vi "StateLED.vi"(0 "Master State In":T1(ring)) -> ()   [LabVIEW 2020]
doc: "This VI manages the apperance of the LEDs. The LED coloration and blink pattern report the robot mode and status. See project documentation for details."
uses:
  <vilib>/Rock Robotics/WPI/DriverStation/WPI_DriverStationRobotMode2.ctl
  GlobalMiscellaneous.vi
  GlobalDriverStationData.vi
  GlobalDrivebase.vi
  GlobalAutonomous.vi
  GlobalPoseAndTargeting.vi
  <vilib>/vision/NI_Vision_Development_Module.lvlib
panel:
  in  "Background":u32(colorbox)=16717311
  in  "Human Control":u32(colorbox)=65280
  in  "Master Caution":u32(colorbox)=16736256
  in  "User Value Choice":u8(slide)=255 step=1 scale=0.0..255.0
  in  "User Saturation Choice":u8(slide)=255 step=1 scale=0.0..255.0
  in  "Pressure Insert":u32(colorbox)=91
  in  "Battery Insert":u32(colorbox)=65282
  in  "Pressure Background":u32(colorbox)=16711680
  in  "Battery Background":u32(colorbox)=16711680
  in  "Pressure LED Length":i32=6
  in  "Battery LED Length":i32=6
  in  "Battery Index":i32=4
  in  "Pressure Index":i32=4
  in  "Swerve 2 LED Index":i32
  in  "Swerve 3 LED Index":i32
  in  "Swerve 0 LED Index":i32=18
  in  "Swerve LED Length":i32=2
  in  "Swerve 1 LED Index":i32=18
  in  "Locate LED":bool
  in  "LED Index":i32
  out "User Blue":u8
  out "User Green":u8=255
  out "User Red":u8
  in  "Choose Hue":bool
  in  "User Hue Choice":u8(slide)=255 step=1 scale=0.0..255.0
  in  "Nominal":u32(colorbox)=65280
  in  "Master Alarm":u32(colorbox)=16711680
  in  "Robot Control":u32(colorbox)=16727040
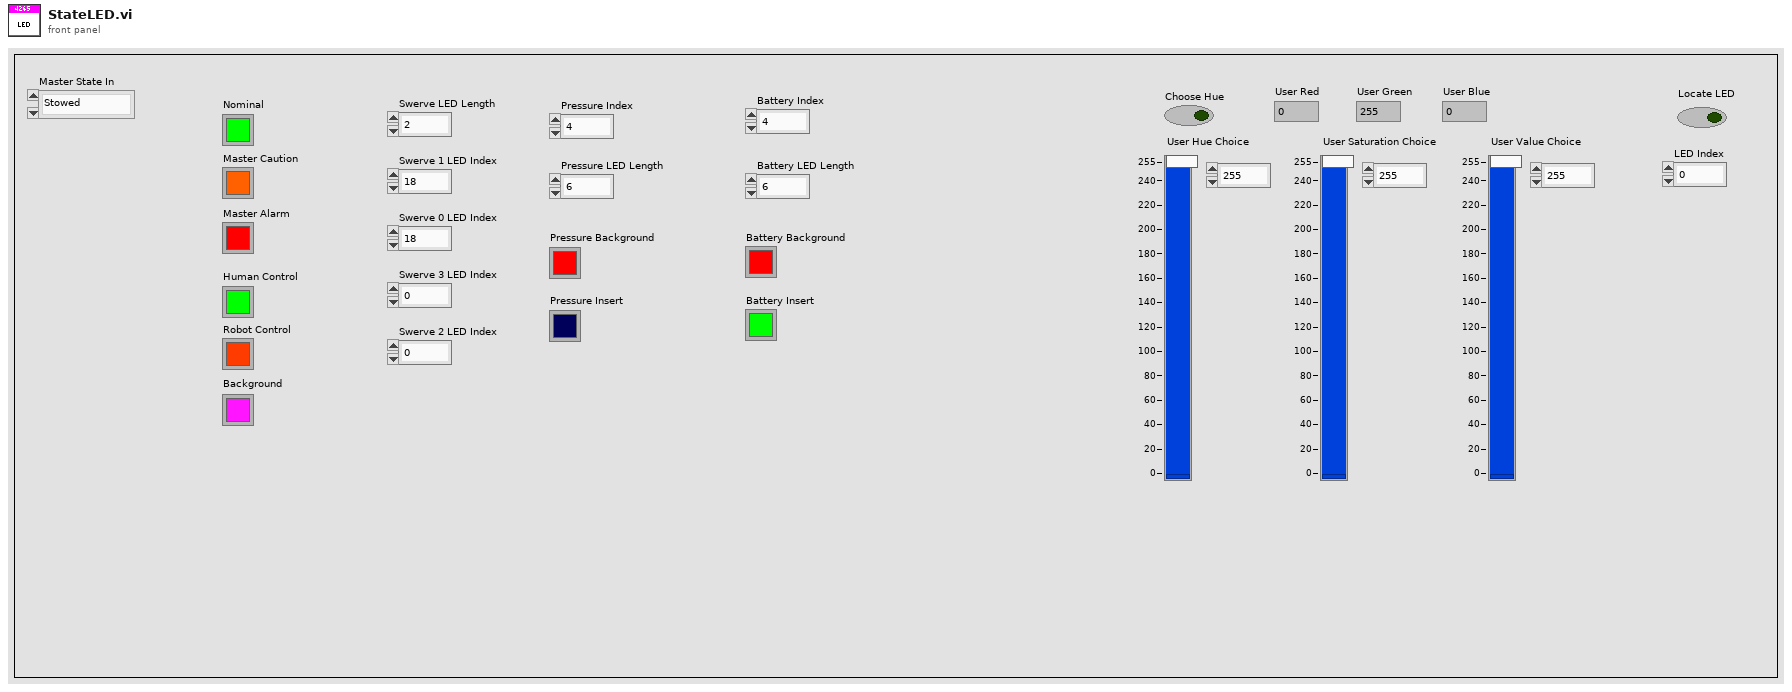
[diagram p1: front panel]
types:
  T1 = enum16{"Stowed", "Balancing", "Scoring", "Hoppering", "Ground", "Shelf"}
  T2 = enum16{"Normal", "Party Mode", "Choose Hue", "Debug", "Locate LED", "Distance Rainbow"}
  T3 = typedef "WPI_DriverStationRobotMode2.ctl" = enum16{"Autonomous Disabled", "Autonomous Enabled", "Teleop Disabled", "Teleop Enabled", "Disconnected", "Finish", "Test Disabled", "Test Enabled", "Emergency Stopped"}
  T4 = enum16{"Low Gear", "High Gear", "Transiting", "Unknown", "Force Low Gear"}
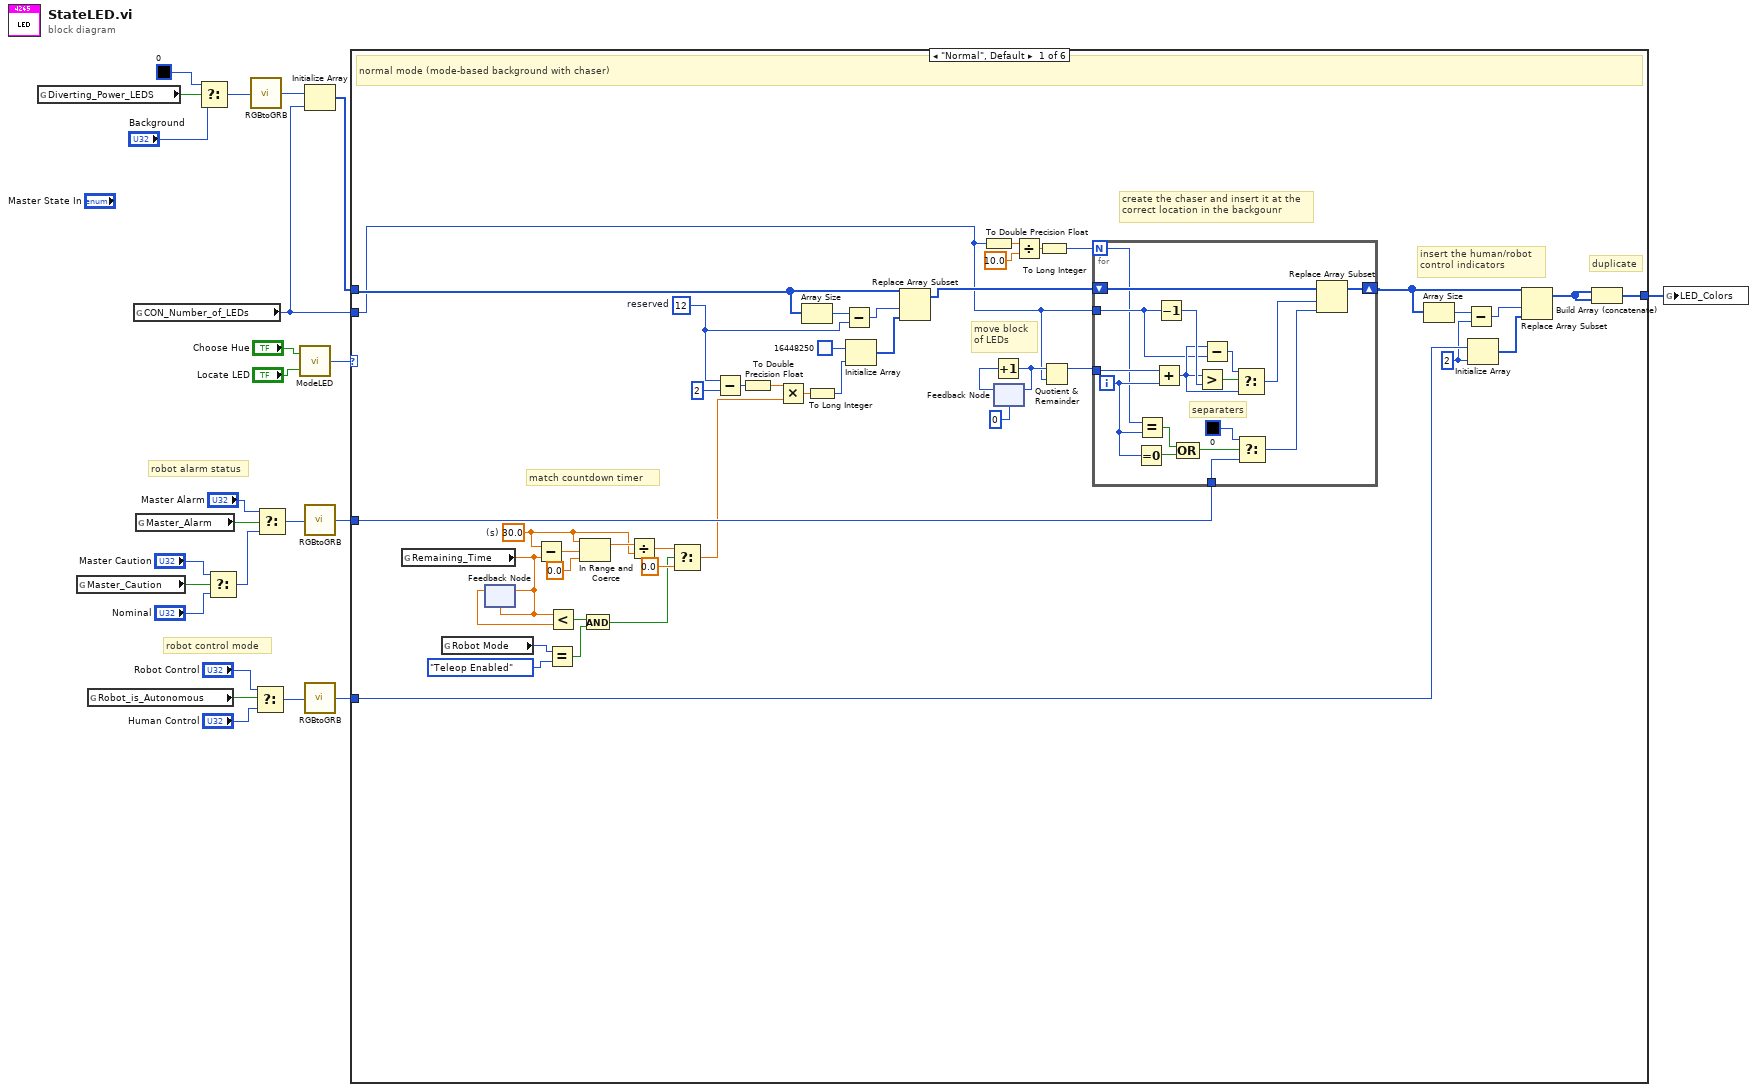
[diagram p0: block diagram]
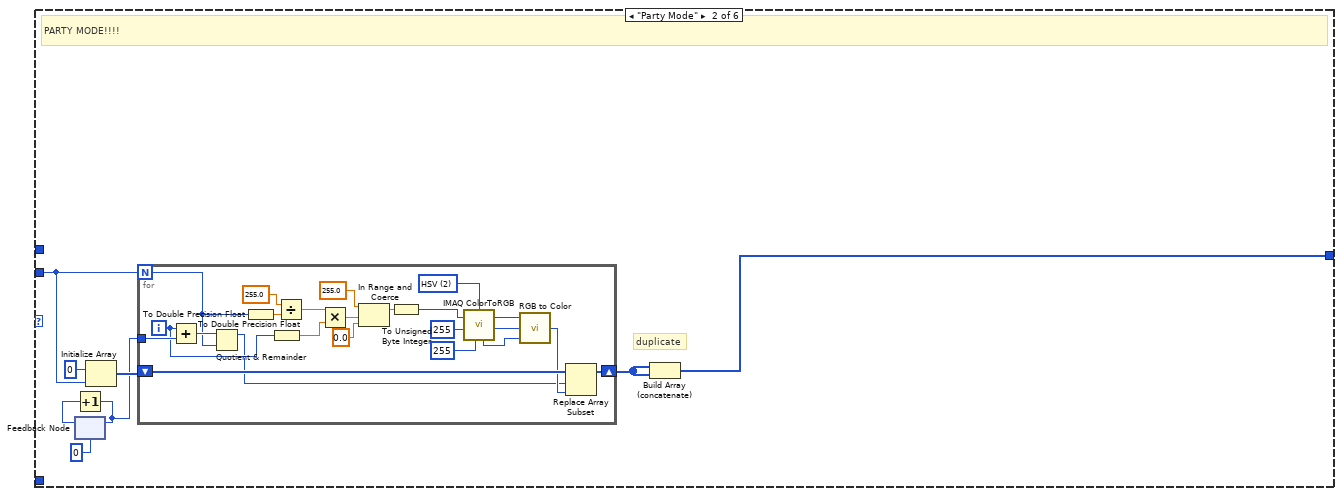
[diagram p2: hidden frame]
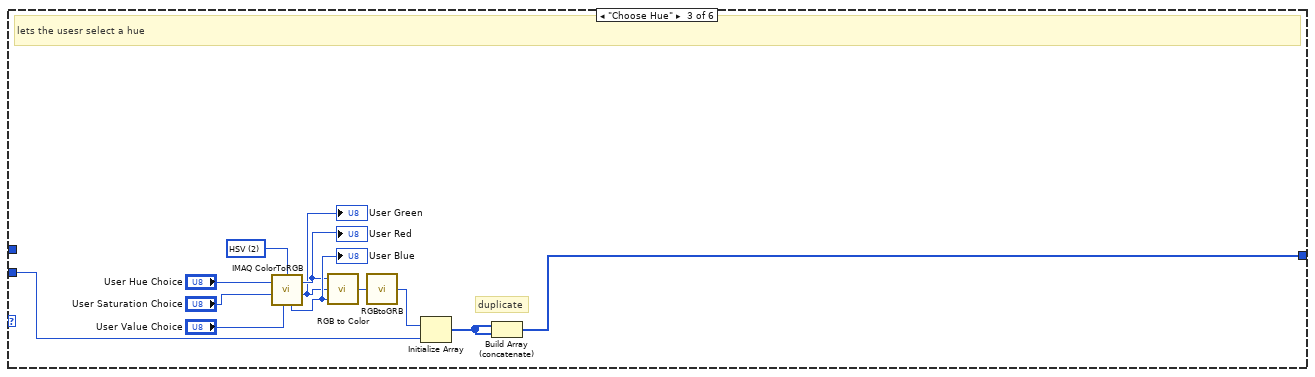
[diagram p3: hidden frame]
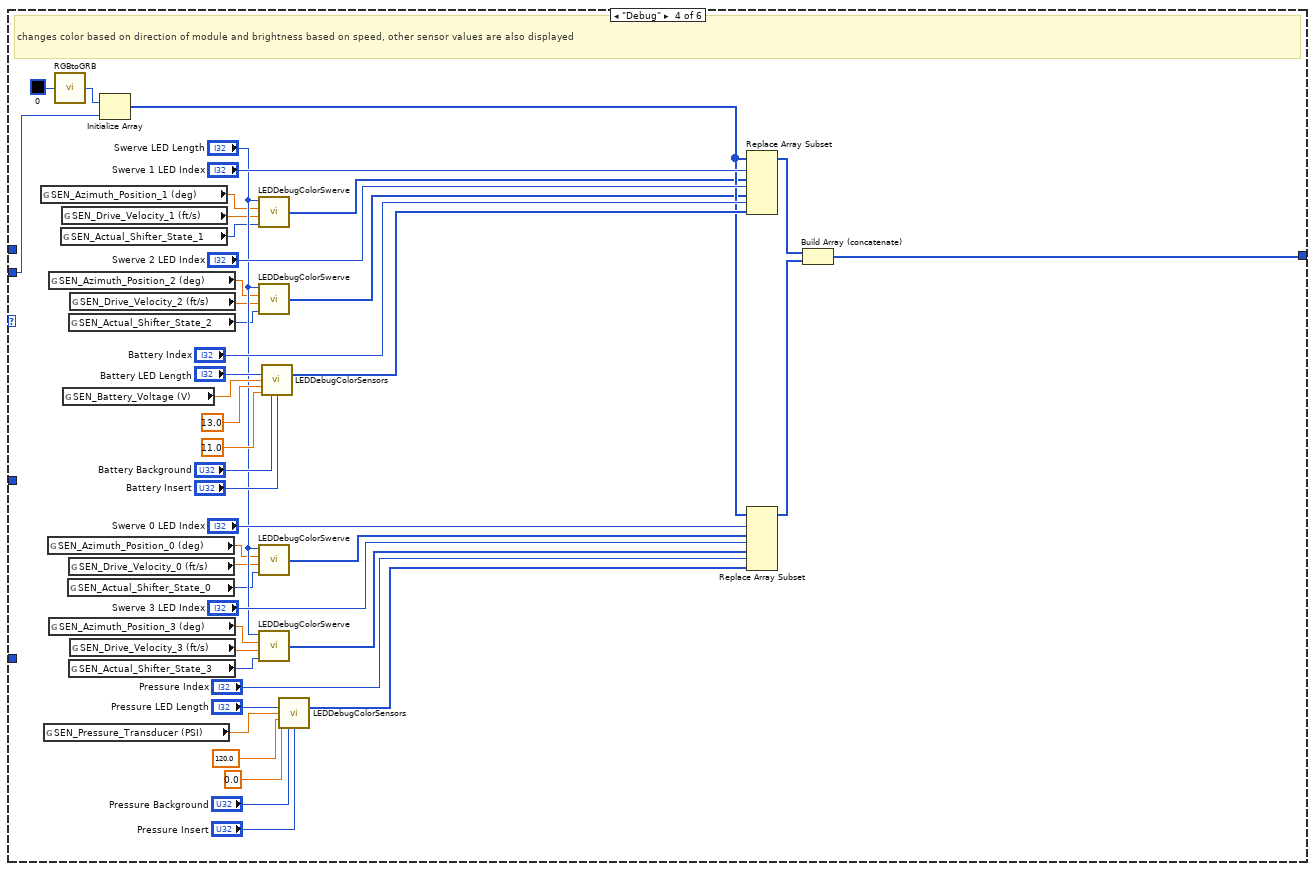
[diagram p4: hidden frame]
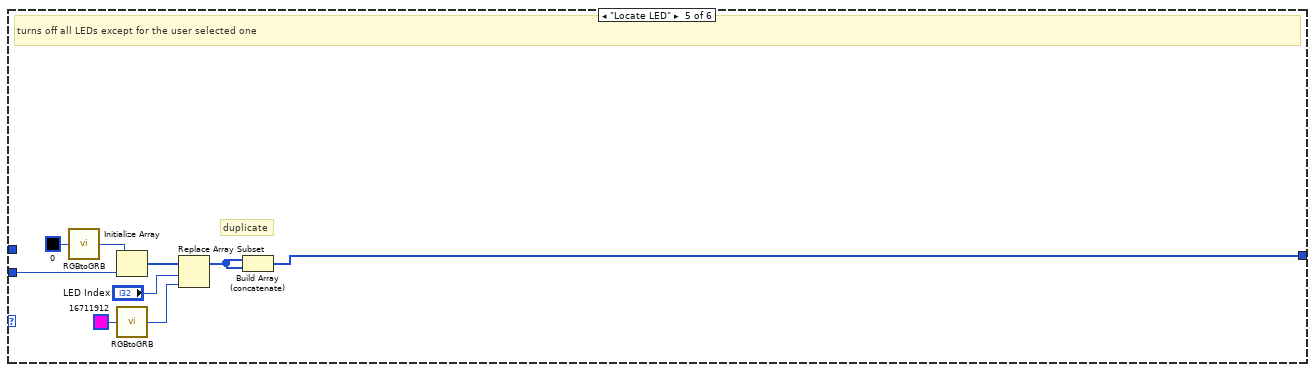
[diagram p5: hidden frame]
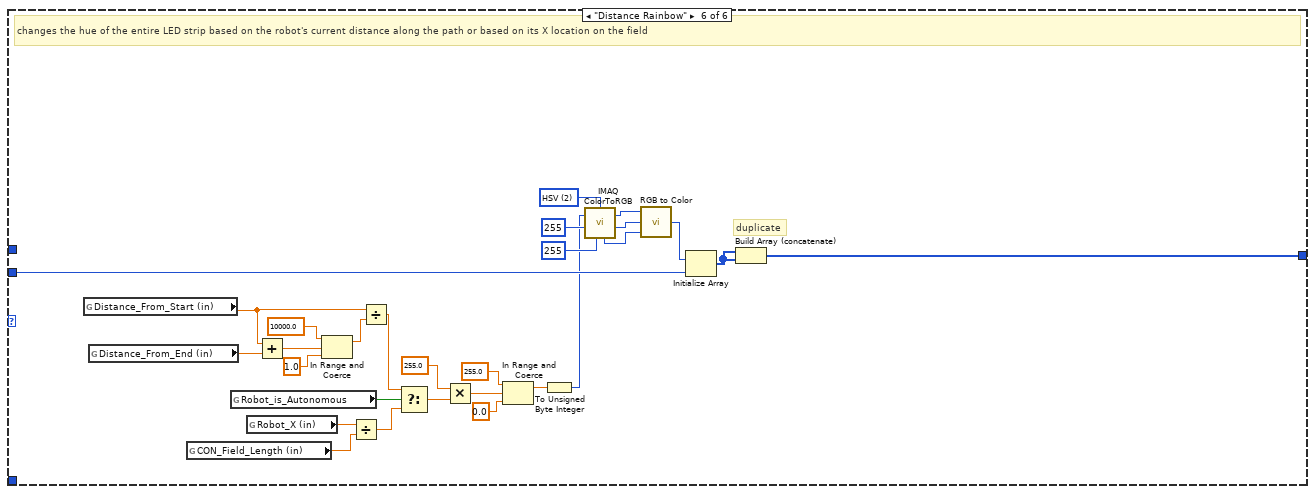
[diagram p6: hidden frame]
diagram:
  # "robot control mode"
  # "robot alarm status"
  n1 = global read "GlobalMiscellaneous.vi" "Diverting_Power_LEDS"() -> (w16:bool)
  n2 = global read "GlobalMiscellaneous.vi" "Master_Caution"() -> (w9:bool)
  n3 = global read "GlobalDriverStationData.vi" "Robot_is_Autonomous"() -> (w14:bool)
  n4 = global read "GlobalMiscellaneous.vi" "CON_Number_of_LEDs"() -> (w1:u16)
  n5 = global read "GlobalMiscellaneous.vi" "Master_Alarm"() -> (w15:bool)
  n6 = Select(t=u32 0 ("Diverting Power"), s=w16, f="Background") -> (s? t:f=w4:u32)
  n7 = Select(t="Master Caution", s=w9, f="Nominal") -> (s? t:f=w8:u32)
  n8 = call "RGBtoGRB.vi"("Color (RGB)"=w4) -> ("Color (GRB)"=w24:u32)
  n9 = Select(t="Robot Control", s=w14, f="Human Control") -> (s? t:f=w13:u32)
  n10 = Select(t="Master Alarm", s=w15, f=w8) -> (s? t:f=w11:u32)
  n11 = call "ModeLED.vi"("Locate LED"="Locate LED", "Choose Hue"="Choose Hue") -> ("LED Mode"=w19:T2)
  n12 = Initialize Array(w24, w1) -> (w21:u32[])
  n13 = call "RGBtoGRB.vi"("Color (RGB)"=w11) -> ("Color (GRB)"=w10:u32)
  n14 = call "RGBtoGRB.vi"("Color (RGB)"=w13) -> ("Color (GRB)"=w20:u32)
  n15 = case shown="\"Normal\", Default" w19 {
    tunnel: w21 -> [w44 _ _ _ _ _]
    tunnel: [w62 w86 w117 w155 w173 w182] -> w3
    tunnel: w20 -> [w68 _ _ _ _ _]
    tunnel: w1 -> [w32 w89 w125 w171 w175 w202]
    tunnel: w10 -> [w35 _ _ _ _ _]
    frame "Normal", Default {
      w53 = 30.0  # (s)
      w46 = 12  # reserved
      w66 = 2 ("dimension size")
      # "create the chaser and insert it at the \ncorrect location in the backgounr"
      # "move block\nof LEDs"
      # "match countdown timer"
      # "duplicate"
      # "insert the human/robot\ncontrol indicators"
      # "normal mode (mode-based background with chaser)"
      n16 = global read "GlobalDriverStationData.vi" "Remaining_Time"() -> (w30:dbl)
      n17 = global read "GlobalDriverStationData.vi" "Robot Mode"() -> (w49:T3)
      n18 = feedback-in #1(w30) -> ()
      n19 = feedback #1(w30) -> (w31:dbl)
      n20 = Subtract(x=w53, y=w30) -> (x-y=w54:dbl)
      n21 = Equal?(x=w49, y=WPI_DriverStationRobotMode2."Teleop Enabled") -> (x = y?=w27:bool)
      n22 = Less?(x=w30, y=w31) -> (x < y?=w29:bool)
      n23 = In Range and Coerce(upper limit=w53, x=w54, lower limit=0.0) -> (coerced(x)=w55:dbl)  [unwired: 1 out]
      n24 = And(x=w29, y=w27) -> (x .and. y?=w28:bool)
      n25 = Divide(x=w55, y=w53) -> (x/y=w52:dbl)
      n26 = Select(t=w52, s=w28, f=0.0) -> (s? t:f=w25:dbl)
      n27 = Subtract(x=w46, y=2) -> (x-y=w47:i32)
      n28 = To Double Precision Float(number=w47) -> (double precision float=w58:dbl)
      n29 = Multiply(x=w58, y=w25) -> (x*y=w57:dbl)
      n30 = Array Size(array=w44) -> (size(s)=w61:i32)
      n31 = To Long Integer(number=w57) -> (32bit integer=w56:i32)
      n32 = Subtract(x=w61, y=w46) -> (x-y=w60:i32)
      n33 = Initialize Array(u32 16448250 ("Color"), w56) -> (w59:u32[])
      n34 = Replace Array Subset(array=w44, new element=w59, index=w60) -> (w33:u32[])
      n35 = To Double Precision Float(number=w32) -> (double precision float=w43:dbl)
      n36 = feedback #2(0) -> (w38:i32)
      n37 = Increment(x=w38) -> (x+1=w37:i32)
      n38 = feedback-in #2(w37) -> ()
      n39 = Divide(x=w43, y=10.0) -> (x/y=w42:dbl)
      n40 = To Long Integer(number=w42) -> (32bit integer=w34:i32)
      n41 = Quotient & Remainder(x=w37, y=w32) -> (x-y*floor(x/y)=w40:i32)  [unwired: 1 out]
      n42 = for {
        N: w34 -> [w69]
        tunnel: w40 -> [w85]
        tunnel: w32 -> [w78]
        shift-right: [w80] -> w36
        shift-left: w33 -> [w81]
        tunnel: w35 -> [w75]
        i -> [w70]
        # "separaters"
        n43 = Equal To 0?(x=w70) -> (x = 0?=w73:bool)
        n44 = Equal?(x=w69, y=w70) -> (x = y?=w71:bool)
        n45 = Add(x=w85, y=w70) -> (x+y=w79:i32)
        n46 = Decrement(x=w78) -> (x-1=w84:u16)
        n47 = Compound Arithmetic op=OR(w71, w73) -> (w72:bool)
        n48 = Greater?(x=w79, y=w84) -> (0:w83:bool)
        n49 = Subtract(x=w79, y=w78) -> (x-y=w77:i32)
        n50 = Select(t=w77, s=w83, f=w79) -> (s? t:f=w82:i32)
        n51 = Select(t=u32 0 ("Color (RGB)"), s=w72, f=w75) -> (s? t:f=w74:u32)
        n52 = Replace Array Subset(array=w81, new element=w74, index=w82) -> (w80:u32[])
      }
      n53 = Array Size(array=w36) -> (size(s)=w67:i32)
      n54 = Subtract(x=w67, y=w66) -> (x-y=w65:i32)
      n55 = Initialize Array(w68, w66) -> (w64:u32[])
      n56 = Replace Array Subset(array=w36, new element=w64, index=w65) -> (w63:u32[])
      n57 = Build Array (concatenate)(w63, w63) -> (w62:u32[])
    }
    frame "Party Mode" {
      # "duplicate"
      # "PARTY MODE!!!!"
      n58 = feedback #3(0) -> (w91:i32)
      n59 = Increment(x=w91) -> (x+1=w88:i32)
      n60 = feedback-in #3(w88) -> ()
      n61 = Initialize Array(u32 0 ("element"), w89) -> (w92:u32[])
      n62 = for {
        N: w89 -> [w96]
        shift-right: [w104] -> w87
        shift-left: w92 -> [w105]
        tunnel: w88 -> [w98]
        i -> [w95]
        w114 = u16 2 items=["RGB", "HSL", "HSV", "HSI"] ("Color Mode")
        n63 = Add(x=w95, y=w98) -> (x+y=w97:i32)
        n64 = Quotient & Remainder(x=w97, y=w96) -> (x-y*floor(x/y)=w94:i32)  [unwired: 1 out]
        n65 = To Double Precision Float(number=w96) -> (double precision float=w113:dbl)
        n66 = To Double Precision Float(number=w95) -> (double precision float=w110:dbl)
        n67 = Divide(x=255.0, y=w113) -> (x/y=w111:dbl)
        n68 = Multiply(x=w111, y=w110) -> (x*y=w109:dbl)
        n69 = In Range and Coerce(upper limit=255.0, x=w109, lower limit=0.0) -> (coerced(x)=w106:dbl)  [unwired: 1 out]
        n70 = To Unsigned Byte Integer(number=w106) -> (unsigned 8bit integer=w99:u8)
        n71 = call "IMAQ ColorToRGB"("Green or Sat value"=u8 255, "Blue or Luma or Val or Inten value"=u8 255, "Red or Hue value"=w99, "Color Mode"=w114) -> ("Blue value"=w100:u8, "Green value"=w101:u8, "Red value"=w102:u8)  [unwired: 1 in, 1 out]
        n72 = call <vilib>:"RGB to Color.vi"("B"=w100, "G"=w101, "R"=w102) -> ("Color"=w103:u32)
        n73 = Replace Array Subset(array=w105, new element=w103, index=w94) -> (w104:u32[])
      }
      n74 = Build Array (concatenate)(w87, w87) -> (w86:u32[])
    }
    frame "Choose Hue" {
      w126 = u16 2 items=["RGB", "HSL", "HSV", "HSI"] ("Color Mode")
      # "duplicate"
      # "lets the usesr select a hue"
      n75 = call "IMAQ ColorToRGB"("Green or Sat value"="User Saturation Choice", "Blue or Luma or Val or Inten value"="User Value Choice", "Red or Hue value"="User Hue Choice", "Color Mode"=w126) -> ("Blue value"=w127:u8, "Green value"=w121:u8, "Red value"=w122:u8)  [unwired: 1 in, 1 out]
      "User Red" <- w122
      "User Green" <- w121
      "User Blue" <- w127
      n76 = call <vilib>:"RGB to Color.vi"("B"=w127, "G"=w121, "R"=w122) -> ("Color"=w120:u32)
      n77 = call "RGBtoGRB.vi"("Color (RGB)"=w120) -> ("Color (GRB)"=w119:u32)
      n78 = Initialize Array(w119, w125) -> (w118:u32[])
      n79 = Build Array (concatenate)(w118, w118) -> (w117:u32[])
    }
    frame "Debug" {
      # "changes color based on direction of module and brightness based on speed, other sensor values are also displayed"
      n80 = global read "GlobalDrivebase.vi" "SEN_Azimuth_Position_1 (deg)"() -> (w140:dbl)
      n81 = global read "GlobalMiscellaneous.vi" "SEN_Pressure_Transducer (PSI)"() -> (w160:dbl)
      n82 = global read "GlobalDrivebase.vi" "SEN_Azimuth_Position_0 (deg)"() -> (w134:dbl)
      n83 = global read "GlobalDrivebase.vi" "SEN_Azimuth_Position_2 (deg)"() -> (w136:dbl)
      n84 = global read "GlobalDrivebase.vi" "SEN_Azimuth_Position_3 (deg)"() -> (w131:dbl)
      n85 = call "RGBtoGRB.vi"("Color (RGB)"=u32 0) -> ("Color (GRB)"=w157:u32)
      n86 = global read "GlobalDrivebase.vi" "SEN_Actual_Shifter_State_1"() -> (w138:T4)
      n87 = global read "GlobalDrivebase.vi" "SEN_Drive_Velocity_1 (ft/s)"() -> (w139:dbl)
      n88 = global read "GlobalMiscellaneous.vi" "SEN_Battery_Voltage (V)"() -> (w159:dbl)
      n89 = global read "GlobalDrivebase.vi" "SEN_Actual_Shifter_State_0"() -> (w132:T4)
      n90 = global read "GlobalDrivebase.vi" "SEN_Actual_Shifter_State_2"() -> (w135:T4)
      n91 = global read "GlobalDrivebase.vi" "SEN_Drive_Velocity_0 (ft/s)"() -> (w133:dbl)
      n92 = global read "GlobalDrivebase.vi" "SEN_Actual_Shifter_State_3"() -> (w129:T4)
      n93 = global read "GlobalDrivebase.vi" "SEN_Drive_Velocity_2 (ft/s)"() -> (w137:dbl)
      n94 = global read "GlobalDrivebase.vi" "SEN_Drive_Velocity_3 (ft/s)"() -> (w130:dbl)
      n95 = Initialize Array(w157, w171) -> (w151:u32[])
      n96 = call "LEDDebugColorSwerve.vi"("Shifter State"=w138, "Drive Velocity (ft/s)"=w139, "Azimuth Angle (deg [-180,180])"=w140, "Swerve LED Length"="Swerve LED Length") -> ("Color Array"=w145:u32[])
      n97 = call "LEDDebugColorSwerve.vi"("Shifter State"=w135, "Drive Velocity (ft/s)"=w137, "Azimuth Angle (deg [-180,180])"=w136, "Swerve LED Length"="Swerve LED Length") -> ("Color Array"=w144:u32[])
      n98 = call "LEDDebugColorSwerve.vi"("Shifter State"=w132, "Drive Velocity (ft/s)"=w133, "Azimuth Angle (deg [-180,180])"=w134, "Swerve LED Length"="Swerve LED Length") -> ("Color Array"=w143:u32[])
      n99 = call "LEDDebugColorSwerve.vi"("Shifter State"=w129, "Drive Velocity (ft/s)"=w130, "Azimuth Angle (deg [-180,180])"=w131, "Swerve LED Length"="Swerve LED Length") -> ("Color Array"=w142:u32[])
      n100 = call "LEDDebugColorSensors.vi"("LED Length"="Battery LED Length", "Value"=w159, "Max"=13.0, "Min"=11.0, "Background Color"="Battery Background", "Color to Insert"="Battery Insert") -> ("Output Color Array"=w152:u32[])  [unwired: 9 in]
      n101 = call "LEDDebugColorSensors.vi"("LED Length"="Pressure LED Length", "Value"=w160, "Max"=120.0, "Min"=0.0, "Background Color"="Pressure Background", "Color to Insert"="Pressure Insert") -> ("Output Color Array"=w146:u32[])  [unwired: 9 in]
      n102 = Replace Array Subset(array=w151, new element #1=w145, index #1="Swerve 1 LED Index", new element #2=w144, index #2="Swerve 2 LED Index", new element #3=w152, index #3="Battery Index") -> (w156:u32[])
      n103 = Replace Array Subset(array=w151, new element #1=w143, index #1="Swerve 0 LED Index", new element #2=w142, index #2="Swerve 3 LED Index", new element #3=w146, index #3="Pressure Index") -> (w150:u32[])
      n104 = Build Array (concatenate)(w156, w150) -> (w155:u32[])
    }
    frame "Locate LED" {
      # "duplicate"
      # "turns off all LEDs except for the user selected one"
      n105 = call "RGBtoGRB.vi"("Color (RGB)"=u32 0) -> ("Color (GRB)"=w180:u32)
      n106 = Initialize Array(w180, w175) -> (w179:u32[])
      n107 = call "RGBtoGRB.vi"("Color (RGB)"=u32 16711912) -> ("Color (GRB)"=w177:u32)
      n108 = Replace Array Subset(array=w179, new element=w177, index="LED Index") -> (w174:u32[])
      n109 = Build Array (concatenate)(w174, w174) -> (w173:u32[])
    }
    frame "Distance Rainbow" {
      w206 = u16 2 items=["RGB", "HSL", "HSV", "HSI"] ("Color Mode")
      # "duplicate"
      # "changes the hue of the entire LED strip based on the robot's current distance along the path or based on its X location on the field"
      n110 = global read "GlobalAutonomous.vi" "Distance_From_Start (in)"() -> (w196:dbl)
      n111 = global read "GlobalAutonomous.vi" "Distance_From_End (in)"() -> (w201:dbl)
      n112 = global read "GlobalPoseAndTargeting.vi" "CON_Field_Length (in)"() -> (w184:dbl)
      n113 = global read "GlobalDriverStationData.vi" "Robot_is_Autonomous"() -> (w185:bool)
      n114 = global read "GlobalPoseAndTargeting.vi" "Robot_X (in)"() -> (w191:dbl)
      n115 = Add(x=w196, y=w201) -> (x+y=w200:dbl)
      n116 = In Range and Coerce(upper limit=10000.0 ("x"), x=w200, lower limit=1.0) -> (coerced(x)=w197:dbl)  [unwired: 1 out]
      n117 = Divide(x=w191, y=w184) -> (x/y=w186:dbl)
      n118 = Divide(x=w196, y=w197) -> (x/y=w195:dbl)
      n119 = Select(t=w195, s=w185, f=w186) -> (s? t:f=w194:dbl)
      n120 = Multiply(x=255.0, y=w194) -> (x*y=w188:dbl)
      n121 = In Range and Coerce(upper limit=255.0 ("x"), x=w188, lower limit=0.0) -> (coerced(x)=w187:dbl)  [unwired: 1 out]
      n122 = To Unsigned Byte Integer(number=w187) -> (unsigned 8bit integer=w192:u8)
      n123 = call "IMAQ ColorToRGB"("Green or Sat value"=u8 255 ("User Saturation Choice 2"), "Blue or Luma or Val or Inten value"=u8 255 ("User Value Choice 2"), "Red or Hue value"=w192, "Color Mode"=w206) -> ("Blue value"=w209:u8, "Green value"=w208:u8, "Red value"=w207:u8)  [unwired: 1 in, 1 out]
      n124 = call <vilib>:"RGB to Color.vi"("B"=w209, "G"=w208, "R"=w207) -> ("Color"=w205:u32)
      n125 = Initialize Array(w205, w202) -> (w183:u32[])
      n126 = Build Array (concatenate)(w183, w183) -> (w182:u32[])
    }
  }
  n127 = global write "GlobalMiscellaneous.vi" "LED_Colors"(w3) -> ()
